vi "PhidgetOpen.vi"(8 "error in":errorcluster, 9 "milliseconds":i32=5000, 10 "Serial Number":i32=-1, 11 "Device In":i32) -> (0 "error out":errorcluster, 1 "Attached?":bool, 2 "Serial Number Return":i32, 3 "Device Out":i32)   [LabVIEW 2014]
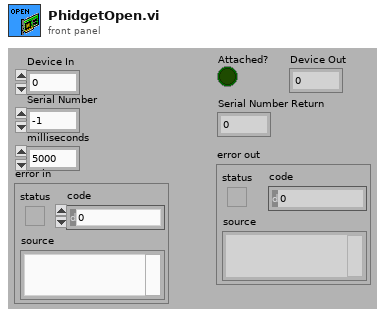
[diagram p1: front panel]
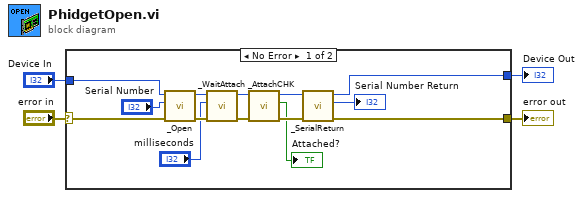
[diagram p0: block diagram]
diagram:
  n1 = case shown="No Error" "error in" {
    selector: "error in" -> [w14 w20]
    tunnel: [w10 w20] -> w3
    tunnel: [w9 w19] -> w2
    tunnel: "Device In" -> [w17 w19]
    frame No Error {
      n2 = call "_Open.vi"("error in"=w14, "Serial Number"="Serial Number", "Device In"=w17) -> ("error out"=w15:errorcluster, "Device Out"=w16:i32)  [unwired: 7 in]
      n3 = call "_WaitAttach.vi"("error in"=w15, "milliseconds"="milliseconds", "Device In"=w16) -> ("error out"=w12:errorcluster, "Device Out"=w13:i32)  [unwired: 7 in]
      n4 = call "_AttachCHK.vi"("error in"=w12, "Device In"=w13) -> ("error out"=w11:errorcluster, "Attached?"=→"Attached?":bool, "Device Out"=w7:i32)  [unwired: 7 in]
      n5 = call "_SerialReturn.vi"("error in"=w11, "Device In"=w7) -> ("error out"=w10:errorcluster, "Serial Number Return"=→"Serial Number Return":i32, "Device Out"=w9:i32)  [unwired: 7 in]
    }
    frame Error {
    }
  }
  "error out" <- w3
  "Device Out" <- w2
